vi "Translator.Translate.Status (Single).vi"(8 "error in (no error)":errorcluster, 9 "Arg":variant, 10 "Msg":T1) -> (0 "error out":errorcluster, 2 "Translated Msg":string)   [LabVIEW 2016]
uses:
  Translator.Message.ctl
  Translator.Global.vi
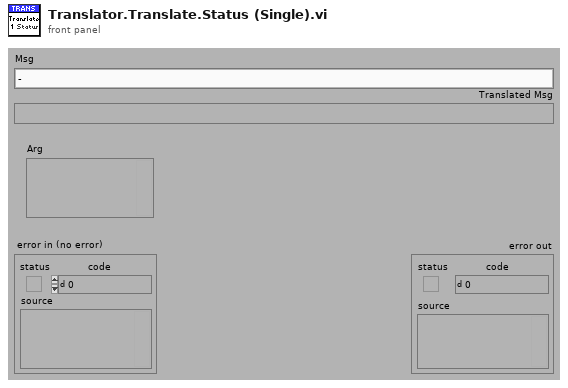
[diagram p1: front panel]
types:
  T1 = typedef "Translator.Message.ctl" = enum16{"-", "Event confirmed", "Log out", "Log in", "Shutdown", "Cancel", "Start", "Continue", "Stop", "On", "Off", "OK", "NOK", "NOK %s", "This", "Prev", "Home", "Work", "In progress...", "Missing", "Empty", "Hardware failure", "Initial", "Error %d >> %s", "Error %d >> %s >> %s", "Starting %s", "Quitting %s", "Configured", "Initializing", "Quitting", "Loading", "Running %s", "Stopped", "Summary", "Do you want to continue?", "Do you want to exit?", "Log out?", "System", "All", "IDLE", "Translating...%s", "Not found", "Alarm %s", "Run", "Skip", "Abort", "Repeat", "Please wait...", "Database disconnected", "Login to database successful", "Login to database failed: %d; %s", "Get process step data for %s", "Changeover off", "Changeover into %s", "Product %s | %s found in cache with status %d at previous station", "Product %s | %s found in database with status %d at previous station", "Product %s | %s not found in cache at previous station", "Product %s | %s not found in database at previous station", "Product %s | %s found in cache with status %d at this station (%d repetion)", "Product %s | %s found in database with status %d at this station (%d repetition)", "Product %s | %s not found in cache at this station", "Product %s | %s not found in database at this station", "Product %s | %s found in cache for component %s | %s", "Product %s | %s found in database for component %s | %s", "Product not found in cache for component %s | %s", "Product not found in database for component %s | %s", "Product %s | %s connected with component %s | %s (cache)", "Product %s | %s connected with component %s | %s (database)", "New data for %s | %s (cache)", "New data for %s | %s (database)", "File %s moved (cache)", "File %s deleted (cache)", "Msg %d >> %s", "PLC LifeBit Failure", "Reconnecting DB", "Reconnecting PLC", "Free disk space is below 1GB - contact technician", "Unable to check product status", "Product %s SN %s checked in DB", "Unable To check status from station %s"}
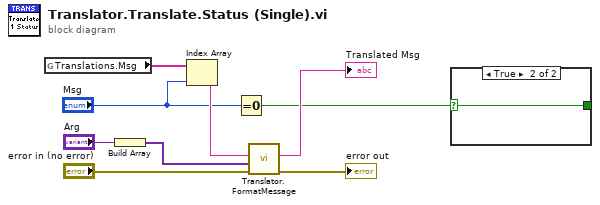
[diagram p0: block diagram]
diagram:
  n1 = global read "Translator.Global.vi" "Translations.Msg"() -> (w7:string[])
  n2 = Build Array("Arg") -> (w3:variant[])
  n3 = Index Array(array=w7, index="Msg") -> (element=w6:string)
  n4 = Equal To 0?(x="Msg") -> (x = 0?=w1:bool)
  n5 = call "Translator.FormatMessage.vi"("error in (no error)"="error in (no error)", "Arguments"=w3, "Msg"=w6) -> ("error out"=→"error out":errorcluster, "Translated Msg"=→"Translated Msg":string)  [unwired: 7 in]
  n6 = case shown="True" w1 {
    selector: w1 -> [w10 w11]
    tunnel: [w10 w11] -> _
    frame False {
    }
    frame True {
    }
  }
